vi "Wrist Flip Requested.vi"(9 "Height Preset":T1=enum."High", 10 "Stored Game Piece":T2, 11 "Operator Buttons":bool[](array[boolean])) -> (3 "Wrist Flip Requested?":bool)   [LabVIEW 2020]
uses:
  manipulator/Implementation/Typedefs/game object.ctl
  manipulator/Implementation/Typedefs/Cascade Height.ctl
  <vilib>/Rock Robotics/WPI/Joystick/XBox Buttons Indexer.ctl
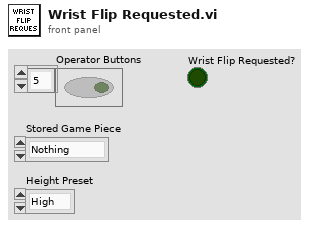
[diagram p1: front panel]
types:
  T1 = typedef "Cascade Height.ctl" = enum16{"Middle", "High"}
  T2 = typedef "game object.ctl" = enum16{"Nothing", "Cone", "Cube"}
  T3 = cluster{"Height Preset":T1, "Stored Game Piece":T2}
  T4 = typedef "XBox Buttons Indexer.ctl" = enum16{"A", "B", "X", "Y", "Left Bumper", "Right Bumper", "Back", "Start", "Left Joystick", "Right Joystick"}
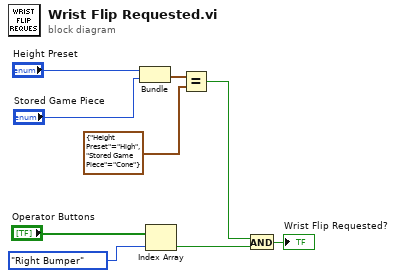
[diagram p0: block diagram]
diagram:
  n1 = Bundle("Height Preset"="Height Preset", "Stored Game Piece"="Stored Game Piece") -> (w3:T3)  [unwired: 1 in]
  n2 = Index Array(array="Operator Buttons", index=XBox_Buttons_Indexer."Right Bumper" ("XBox Buttons")) -> (element=w4:bool)
  n3 = Equal?(x=w3, y=T3 {"Height Preset"=enum."High", "Stored Game Piece"=enum."Cone"}) -> (x = y?=w1:bool)
  n4 = And(x=w1, y=w4) -> (x .and. y?=→"Wrist Flip Requested?":bool)
